vi "CamTest.vi"() -> ()   [LabVIEW 2011]
uses:
  <vilib>/Rock Robotics/WPI/Camera/WPI_CameraImageSize.ctl
  <vilib>/vision/Image Controls.llb/IMAQ Image.ctl
  Vision Code/CameraImageGlobal.vi
panel:
  out "Number of Targets":i32(knob) scale=0.0..5.0
  in  "Margin of Error":i32=25
  in  "Draw Targets":bool
  out "Processing Time":cluster{u32}(graph)
  out "Distance":T1(array[cluster])
  in  "stop":bool
  out "Image Out R":T2(plugin-control)
  out "Image Out L":T2(plugin-control)
  in  "Image Size":T3
  in  "compression":i32
  in  "fps":i32=30
  out "Startup Time":u32
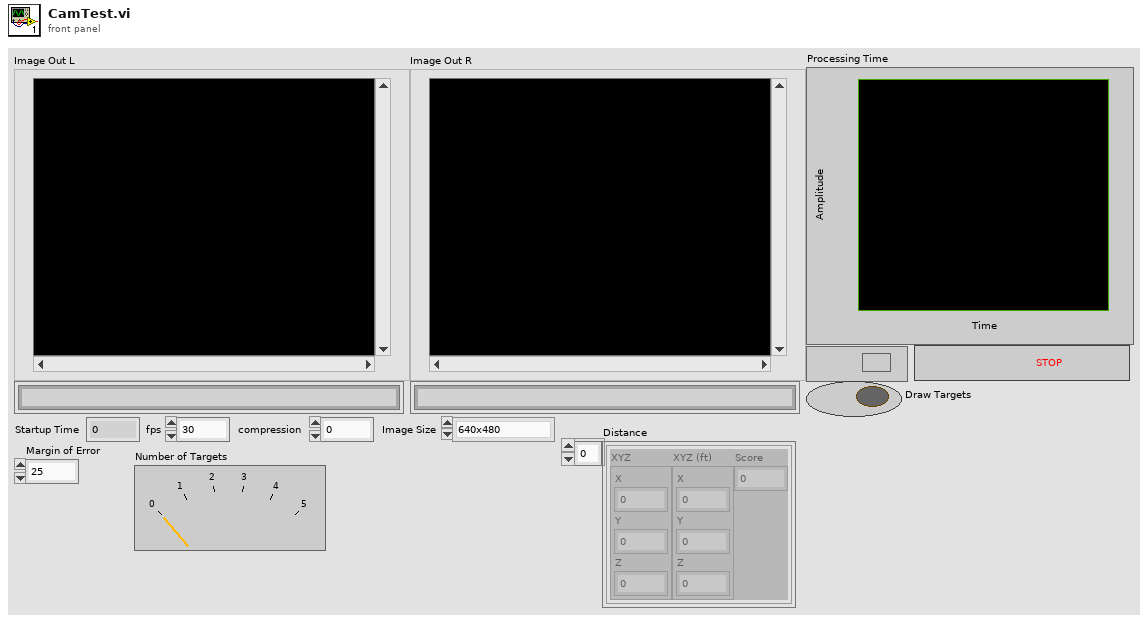
[diagram p1: front panel]
types:
  T1 = cluster{"XYZ":cluster{"X":dbl, "Y":dbl, "Z":dbl}, "XYZ (ft)":cluster{"X":dbl, "Y":dbl, "Z":dbl}, "Score":dbl}[]
  T2 = typedef "IMAQ Image.ctl" = refnum<image>
  T3 = typedef "WPI_CameraImageSize.ctl" = enum16{"640x480", "320x240", "160x120"}
  T4 = cluster{"fps":i32, "compression":i32, "Image Size":T3}
  T5 = typedef "Image Type" = u32
  T6 = cluster{"address":string, "New Image":T2, "New Image":T2, "Camera Settings":cluster{"fps":i32, "compression":i32, "Image Size":T3}}
  T7 = cluster{"Center of Mass":cluster{"X":dbl, "Y":dbl}, "First Pixel":cluster{"X":dbl, "Y":dbl}, "Bounding Rect":cluster{"Left":dbl, "Top":dbl, "Right":dbl, "Bottom":dbl}, "Bounding Rect Size":cluster{"X":dbl, "Y":dbl}, "Area":dbl}[]
  T8 = cluster{"Start Point":cluster{"X":sgl, "Y":sgl}, "End Point":cluster{"X":sgl, "Y":sgl}, "Length":dbl, "Orientation":dbl, "Score":dbl}[]
  T9 = cluster{"LeftImage_Mark":cluster{"Blob":cluster{"Center of Mass":cluster{"X":dbl, "Y":dbl}, "First Pixel":cluster{"X":dbl, "Y":dbl}, "Bounding Rect":cluster{"Left":dbl, "Top":dbl, "Right":dbl, "Bottom":dbl}, "Bounding Rect Size":cluster{"X":dbl, "Y":dbl}, "Area":dbl}, "Cluster":cluster{"TopLeft":cluster{"X":dbl, "Y":dbl}, "TopRight":cluster{"X":dbl, "Y":dbl}, "BottomRight":cluster{"X":dbl, "Y":dbl}, "BottomLeft":cluster{"X":dbl, "Y":dbl}}}, "RightImage_Mark":cluster{"Blob":cluster{"Center of Mass":cluster{"X":dbl, "Y":dbl}, "First Pixel":cluster{"X":dbl, "Y":dbl}, "Bounding Rect":cluster{"Left":dbl, "Top":dbl, "Right":dbl, "Bottom":dbl}, "Bounding Rect Size":cluster{"X":dbl, "Y":dbl}, "Area":dbl}, "Cluster":cluster{"TopLeft":cluster{"X":dbl, "Y":dbl}, "BottomRight":cluster{"X":dbl, "Y":dbl}, "BottomLeft":cluster{"X":dbl, "Y":dbl}, "TopRight":cluster{"X":dbl, "Y":dbl}}}, "Numeric Control":dbl}[]
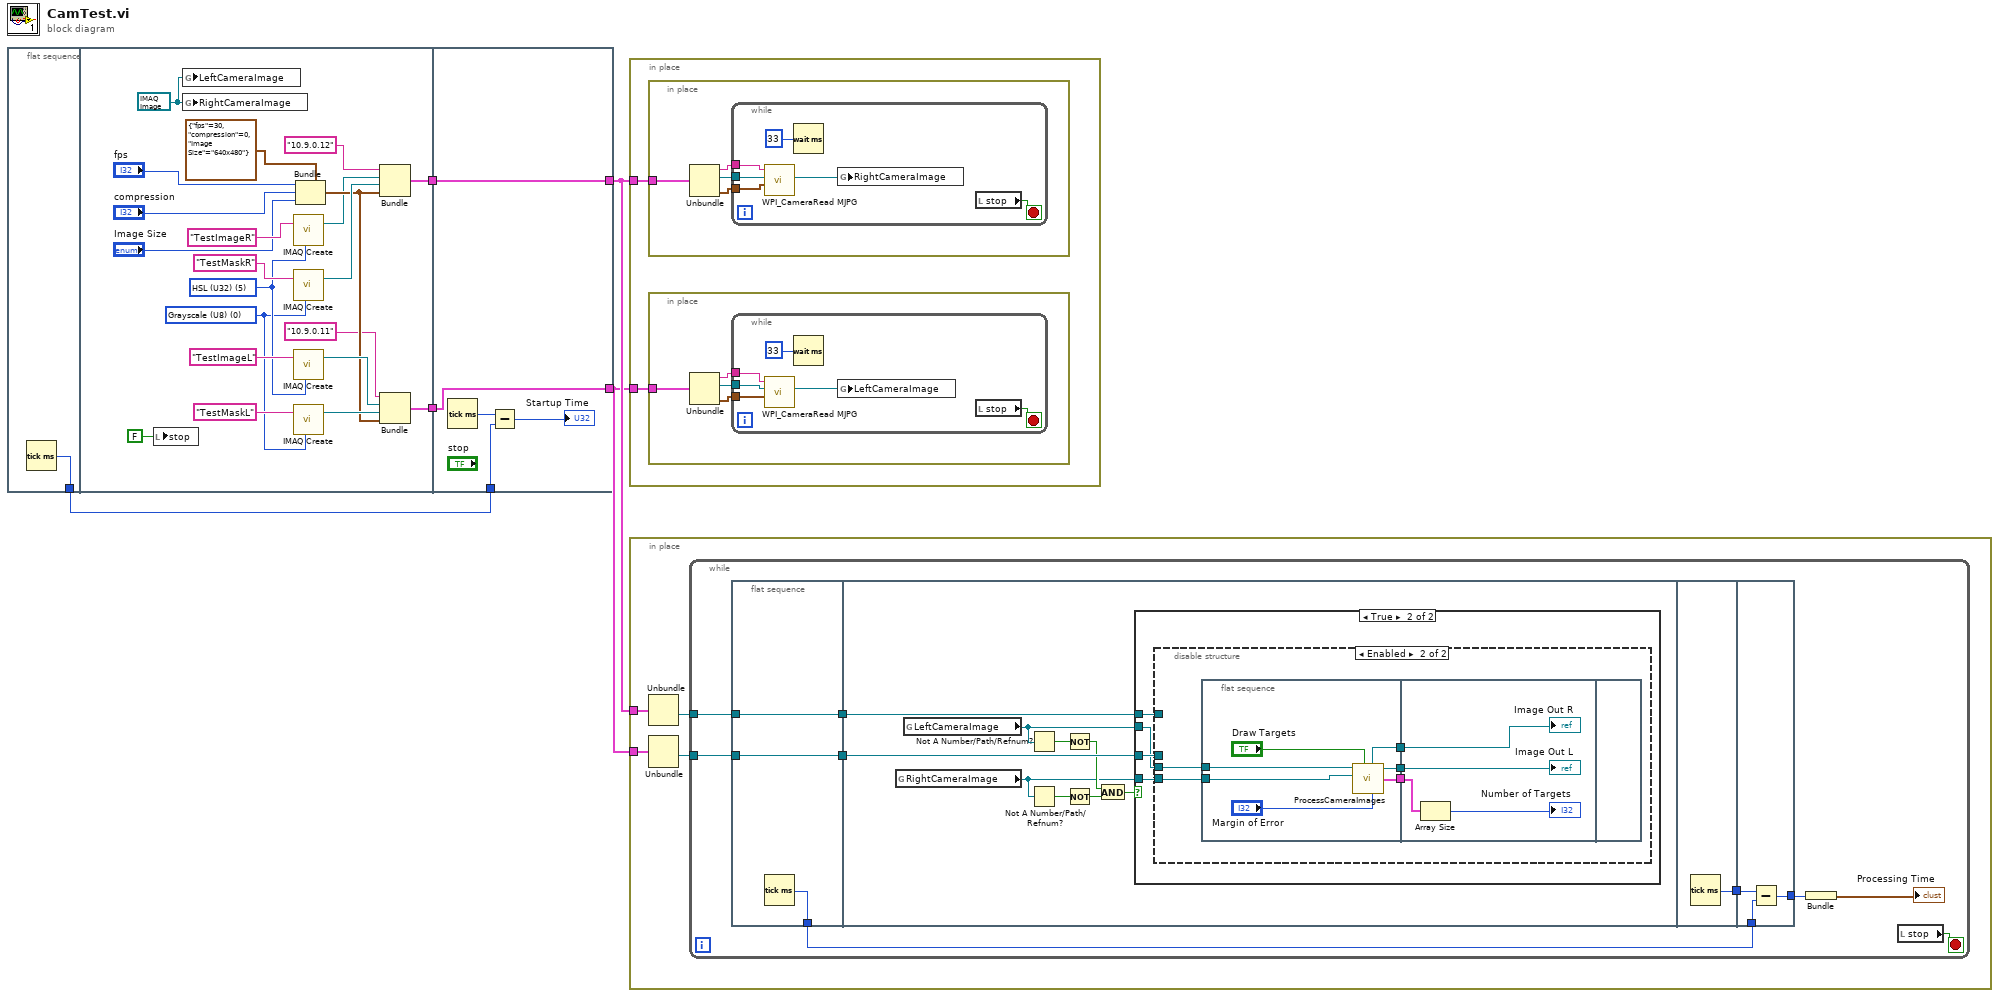
[diagram p0: block diagram]
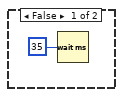
[diagram p2: hidden frame]
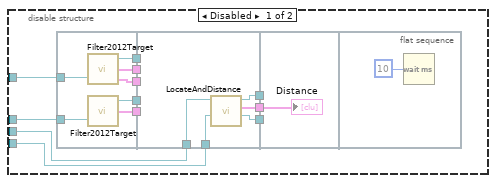
[diagram p3: hidden frame]
diagram:
  n1 = flat-sequence {
    tunnel: [w6] -> w3
    tunnel: [w8] -> w5
    tunnel: [w7] -> w4
    tunnel: [w31] -> w2
    tunnel: [w32] -> w1
    tunnel: w5 -> [w32]
    tunnel: w4 -> [w31]
    tunnel: w3 -> [w30]
    frame #0 {
      n2 = Tick Count (ms)() -> (millisecond timer value=w6:u32)
    }
    frame #1 {
      w9 = T2 refnum ("LeftCameraImage")
      w10 = T5 0 items=["Grayscale (U8)", "Grayscale (I16)", "Grayscale (SGL)", "Complex (CSG)", "RGB (U32)", "HSL (U32)", "RGB (U64)", "Grayscale (U16)"] ("Image Type")
      w11 = T5 5 items=["Grayscale (U8)", "Grayscale (I16)", "Grayscale (SGL)", "Complex (CSG)", "RGB (U32)", "HSL (U32)", "RGB (U64)", "Grayscale (U16)"] ("Image Type")
      n3 = local write "stop"(FALSE ("stop")) -> ()
      n4 = global write "CameraImageGlobal.vi" "LeftCameraImage"(w9) -> ()
      n5 = global write "CameraImageGlobal.vi" "RightCameraImage"(w9) -> ()
      n6 = call "IMAQ Create"("Image Name"="TestImageR", "Image Type"=w11) -> ("New Image"=w12:T2)  [unwired: 3 in, 1 out]
      n7 = call "IMAQ Create"("Image Name"="TestMaskR", "Image Type"=w10) -> ("New Image"=w21:T2)  [unwired: 3 in, 1 out]
      n8 = call "IMAQ Create"("Image Name"="TestImageL", "Image Type"=w11) -> ("New Image"=w23:T2)  [unwired: 3 in, 1 out]
      n9 = call "IMAQ Create"("Image Name"="TestMaskL", "Image Type"=w10) -> ("New Image"=w22:T2)  [unwired: 3 in, 1 out]
      n10 = Bundle(cluster=T4 {"fps"=30, "compression"=0, "Image Size"=enum."640x480"} ("Camera Settings"), "fps"="fps", "compression"="compression", "Image Size"="Image Size") -> (w17:T4)
      n11 = Bundle("address"="10.9.0.12", "New Image"=w12, "New Image"=w21, "Camera Settings"=w17) -> (w7:T6)  [unwired: 1 in]
      n12 = Bundle("address"="10.9.0.11", "New Image"=w23, "New Image"=w22, "Camera Settings"=w17) -> (w8:T6)  [unwired: 1 in]
    }
    frame #2 {
      n13 = Tick Count (ms)() -> (millisecond timer value=w29:u32)
      n14 = Subtract(x=w29, y=w30) -> (x-y=→"Startup Time":u32)
    }
  }
  n15 = in-place {
    in-place-border: w2 -> [w34]
    in-place-border: w1 -> [w33]
    n16 = in-place {
      in-place-border: w34 -> [w35]
      n17 = Unbundle(w35) -> ("address"=w38:string, "New Image"=w37:T2, "Camera Settings"=w36:T4)  [unwired: 1 out]
      n18 = while {
        tunnel: w38 -> [w42]
        tunnel: w37 -> [w41]
        tunnel: w36 -> [w40]
        stop <- w44 stop-if-true
        n19 = call <vilib>:"WPI_CameraRead MJPG.vi"("Camera Settings"=w40, "Image"=w41, "address"=w42) -> ("Image Out"=w39:T2)  [unwired: 7 in, 1 out]
        n20 = Wait (ms)(milliseconds to wait=u32 33) -> ()  [unwired: 1 out]
        n21 = global write "CameraImageGlobal.vi" "RightCameraImage"(w39) -> ()
        n22 = local read "stop"() -> (w44:bool)
      }
    }
    n23 = in-place {
      in-place-border: w33 -> [w48]
      n24 = Unbundle(w48) -> ("address"=w47:string, "New Image"=w46:T2, "Camera Settings"=w45:T4)  [unwired: 1 out]
      n25 = while {
        tunnel: w47 -> [w52]
        tunnel: w46 -> [w51]
        tunnel: w45 -> [w50]
        stop <- w54 stop-if-true
        n26 = call <vilib>:"WPI_CameraRead MJPG.vi"("Camera Settings"=w50, "Image"=w51, "address"=w52) -> ("Image Out"=w49:T2)  [unwired: 7 in, 1 out]
        n27 = Wait (ms)(milliseconds to wait=u32 33) -> ()  [unwired: 1 out]
        n28 = global write "CameraImageGlobal.vi" "LeftCameraImage"(w49) -> ()
        n29 = local read "stop"() -> (w54:bool)
      }
    }
  }
  n30 = in-place {
    in-place-border: w2 -> [w58]
    in-place-border: w1 -> [w57]
    n31 = Unbundle(w58) -> ("New Image"=w55:T2)  [unwired: 3 out]
    n32 = Unbundle(w57) -> ("New Image"=w56:T2)  [unwired: 3 out]
    n33 = while {
      tunnel: w56 -> [w67]
      tunnel: w55 -> [w66]
      stop <- w65 stop-if-true
      n34 = flat-sequence {
        tunnel: w66 -> [w69]
        tunnel: w67 -> [w70]
        tunnel: [w70] -> w64
        tunnel: [w69] -> w63
        tunnel: [w68] -> w62
        tunnel: w64 -> [w79]
        tunnel: w63 -> [w78]
        tunnel: [w129] -> w61
        tunnel: w62 -> [w131]
        tunnel: w61 -> [w130]
        tunnel: [w132] -> w60
        frame #0 {
          n35 = Tick Count (ms)() -> (millisecond timer value=w68:u32)
        }
        frame #1 {
          n36 = global read "CameraImageGlobal.vi" "RightCameraImage"() -> (w71:T2)
          n37 = global read "CameraImageGlobal.vi" "LeftCameraImage"() -> (w72:T2)
          n38 = Not A Number/Path/Refnum?(number/path/refnum=w72) -> (NaN/Path/Refnum?=w76:bool)
          n39 = Not A Number/Path/Refnum?(number/path/refnum=w71) -> (NaN/Path/Refnum?=w77:bool)
          n40 = Not(x=w76) -> (.not. x?=w75:bool)
          n41 = Not(x=w77) -> (.not. x?=w74:bool)
          n42 = And(x=w75, y=w74) -> (x .and. y?=w73:bool)
          n43 = case shown="True" w73 {
            tunnel: w79 -> [_ w84]
            tunnel: w78 -> [_ w83]
            tunnel: w72 -> [_ w82]
            tunnel: w71 -> [_ w81]
            frame False {
              n44 = Wait (ms)(milliseconds to wait=u32 35) -> ()  [unwired: 1 out]
            }
            frame True {
              n45 = disable-structure shown="Enabled" {
                disable-tunnel: w84 -> [w88 _]
                disable-tunnel: w83 -> [w87 _]
                disable-tunnel: w82 -> [w86 w117]
                disable-tunnel: w81 -> [w85 w116]
                frame Disabled {
                  n46 = flat-sequence {
                    tunnel: w87 -> [w103]
                    tunnel: w88 -> [w101]
                    tunnel: [w100] -> w96
                    tunnel: [w102] -> w95
                    tunnel: [w99] -> w94
                    tunnel: [w98] -> w93
                    tunnel: [w97] -> w92
                    tunnel: w96 -> [_]
                    tunnel: w95 -> [_]
                    tunnel: [w108] -> w91
                    tunnel: [w107] -> w90
                    tunnel: [w106] -> w89
                    tunnel: w94 -> [_]
                    tunnel: w93 -> [_]
                    tunnel: w92 -> [_]
                    tunnel: w86 -> [w105]
                    tunnel: w85 -> [w104]
                    tunnel: w91 -> [w111]
                    tunnel: w90 -> [w110]
                    tunnel: w89 -> [w109]
                    frame #0 {
                      n47 = call "Filter2012Target.vi"("Image Dst"=w103) -> ("Image Out"=w99:T2, "Blob Array"=w102:T7, "Lines Calibrated"=w97:T8)  [unwired: 1 in]
                      n48 = call "Filter2012Target.vi"("Image Dst"=w101) -> ("Image Out"=w98:T2, "Blob Array"=w100:T7)  [unwired: 1 in, 1 out]
                    }
                    frame #1 {
                      n49 = call "LocateAndDistance.vi"("ImageR In"=w104, "ImageL In"=w105) -> ("ImageR Out"=w107:T2, "Distance"=w106:T1, "ImageL Out"=w108:T2)  [unwired: 2 in, 1 out]
                    }
                    frame #2 {
                      "Distance" <- w109
                    }
                    frame #3 {
                      n50 = Wait (ms)(milliseconds to wait=u32 10) -> ()  [unwired: 1 out]
                    }
                  }
                }
                frame Enabled {
                  n51 = flat-sequence {
                    tunnel: w117 -> [w124]
                    tunnel: w116 -> [w123]
                    tunnel: [w122] -> w115
                    tunnel: [w121] -> w114
                    tunnel: [w118] -> w113
                    tunnel: w115 -> [w128]
                    tunnel: w114 -> [w127]
                    tunnel: w113 -> [w126]
                    frame #0 {
                      n52 = call "ProcessCameraImages.vi"("Margin of Error"="Margin of Error", "Draw Targets"="Draw Targets", "R_Image"=w123, "L_Image"=w124) -> ("TargetMatch"=w118:T9, "L_Image Out"=w122:T2, "R_Image Out"=w121:T2)  [unwired: 3 in, 1 out]
                    }
                    frame #1 {
                      n53 = Array Size(array=w126) -> (size(s)=→"Number of Targets":i32)
                      "Image Out L" <- w128
                      "Image Out R" <- w127
                    }
                    frame #2 {
                    }
                  }
                }
              }
            }
          }
        }
        frame #2 {
          n54 = Tick Count (ms)() -> (millisecond timer value=w129:u32)
        }
        frame #3 {
          n55 = Subtract(x=w130, y=w131) -> (x-y=w132:u32)
        }
      }
      n56 = Bundle(w60) -> (→"Processing Time":cluster{u32})  [unwired: 1 in]
      n57 = local read "stop"() -> (w65:bool)
    }
  }
